vi "timed-delay-example.vi"() -> ()   [LabVIEW 2020]
uses:
  <vilib>/Platform/TimedLoop/XDataNode/timing_clust.ctl
  <vilib>/Platform/TimedLoop/XDataNode/nitl_modes.ctl
  <vilib>/Platform/TimedLoop/XDataNode/wakeup.ctl
  <vilib>/platform/TimedLoop/XDataNode/XDataNode.xnode
  <vilib>/Platform/TimedLoop/XDataNode/XDNodeRunTimeDep.lvlib
  <vilib>/measure/NI_MABase.lvlib
panel:
  out "Error out":errorcluster
  in  "Error":errorcluster
  out "Frame Duration":dbl
  in  "Delay between graphs(s)":dbl=1.0
  out "Waveform Graph":waveform(dbl)(graph)
  in  "Duration (s)":dbl=10.0
  in  "Samping rate (Sample/s)":dbl=10000.0
  in  "Frequency (Hz)":dbl=1000.0
  in  "Amplitude":dbl=1.0
  out "Waveform Graph":waveform(dbl)(graph)
  in  "Duration (s)":dbl=5.0
  in  "Samping rate (Sample/s)":dbl=1000.0
  in  "Frequency (Hz)":dbl=100.0
  in  "Amplitude":dbl=2.0
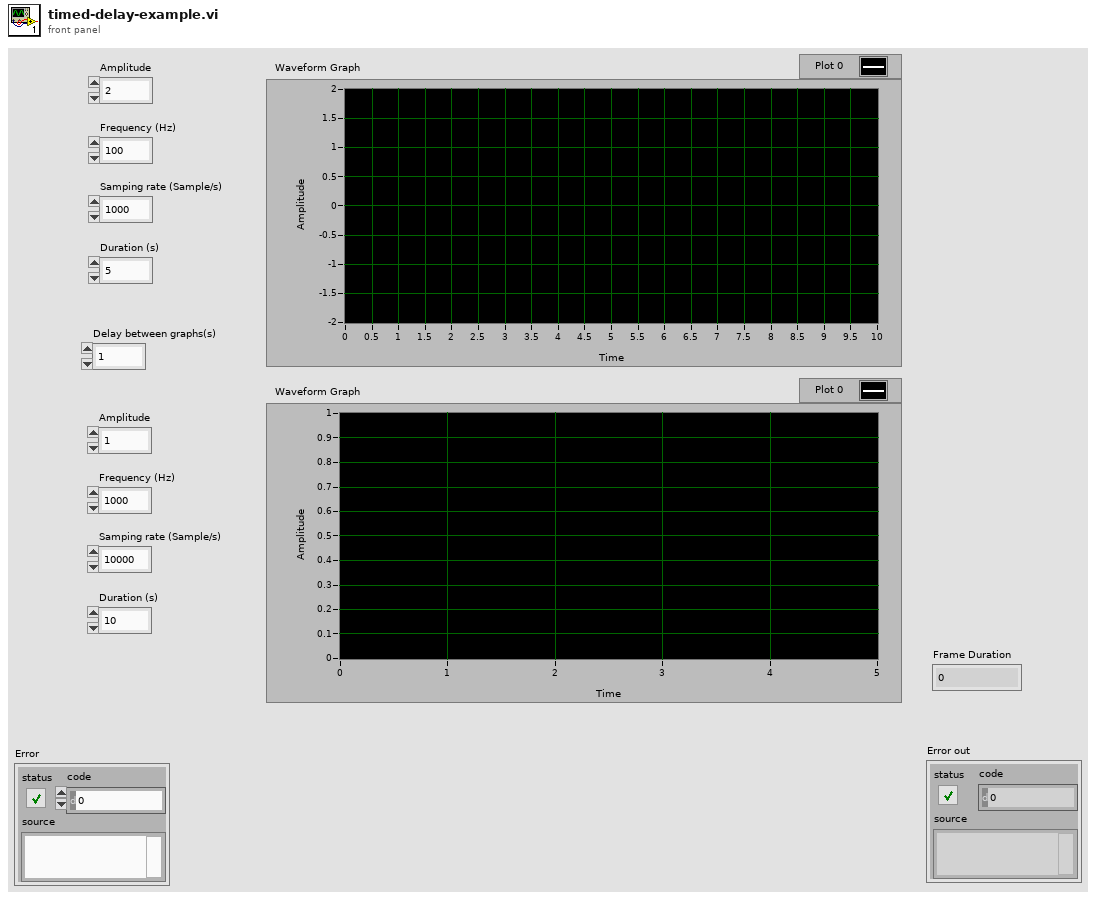
[diagram p1: front panel]
types:
  T1 = typedef "XDNodeRunTimeDep.lvlib/timing_clust.ctl" = cluster{"Expected End [f-1]":u64, "Actual End [f-1]":u64, "Finished Late? [f-1]":bool, "Expected End [i-1]":u64, "Actual End [i-1]":u64, "Finished Late? [i-1]":bool, "Expected Start [i]":u64, "Actual Start [i]":u64, "Expected Start [f]":u64, "Actual Start [f]":u64, "Source Name":string, "Structure Name":string, "Period":i64, "Deadline":i64, "Offset":i64, "Start":i64, "Priority":i32, "Timeout":i32, "Mode":T2, "Wakeup Reason":T3, "Error":errorcluster, "Source Type":string, "Secondary Source Type":string, "Global End Time":u64, "Global Start Time":u64, "Frame Duration":u64, "Iteration Duration":u64, "Assigned CPU":i32, "I/O Scan Engine Mode":u32}
  T2 = typedef "XDNodeRunTimeDep.lvlib/nitl_modes.ctl" = enum32{"No Change", "Process missed periods, maintain original phase", "Discard missed periods, maintain original phase", "Process missed periods, ignore original phase", "Discard missed periods, ignore original phase"}
  T3 = typedef "XDNodeRunTimeDep.lvlib/wakeup.ctl" = enum32{"Normal", "Aborted", "Asynchronous wakeup", "Timing source error", "Timed loop error", "Timeout"}
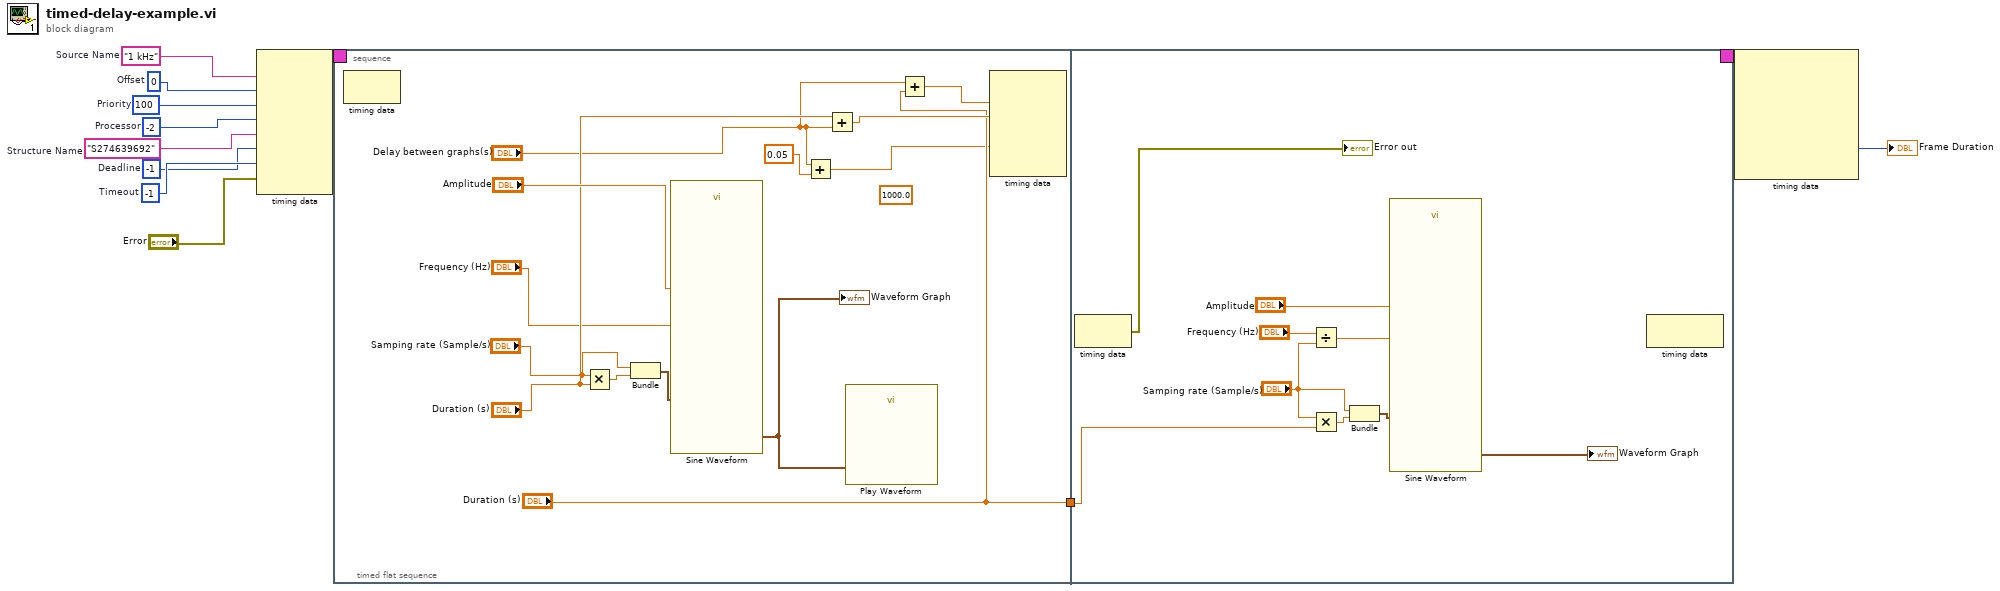
[diagram p0: block diagram]
diagram:
  w1 = "S274639692"  # Structure Name
  w2 = -2  # Processor
  w3 = 100  # Priority
  w4 = i64 0  # Offset
  w5 = "1 kHz"  # Source Name
  w6 = i64 -1  # Deadline
  w7 = -1  # Timeout
  n1 = node-c288(w5, w4, w3, w2, w1, w6, w7, "Error") -> (w11:T1)
  n2 = timed-sequence {
    timing: w11 -> [_]
    timing-out: [_] -> w10
    n3 = timed-flat-sequence {
      tunnel: ["Duration (s)"] -> w12
      tunnel: w12 -> [w34]
      frame #0 {
        (unwired) 1000.0 ("y")
        n4 = node-c288() -> ()  [unwired: 1 in, 1 out]
        n5 = Multiply(x="Samping rate (Sample/s)", y="Duration (s)") -> (x*y=w24:dbl)
        n6 = Bundle("Samping rate (Sample/s)"="Samping rate (Sample/s)", w24) -> (w25:cluster{"Samping rate (Sample/s)":dbl, dbl})  [unwired: 1 in]
        n7 = call <vilib>:"Sine Waveform.vi"("sampling info"=w25, "amplitude"="Amplitude", "frequency"="Frequency (Hz)") -> ("signal out"=w22:waveform(dbl))  [unwired: 7 in, 1 out]
        "Waveform Graph" <- w22
        n8 = Add(x="Delay between graphs(s)", y=0.05) -> (x+y=w14:dbl)
        n9 = Add(x="Duration (s)", y="Delay between graphs(s)") -> (x+y=w19:dbl)
        n10 = call "Play Waveform"("Data"=w22) -> ()  [unwired: 18 in, 1 out]
        n11 = Add(x="Delay between graphs(s)", y="Duration (s)") -> (x+y=w16:dbl)
        n12 = node-c288(w16, w19, w14) -> ()  [unwired: 3 in, 1 out]
      }
      frame #1 {
        n13 = node-c288() -> (→"Error out":errorcluster)  [unwired: 1 in]
        n14 = Divide(x="Frequency (Hz)", y="Samping rate (Sample/s)") -> (x/y=w36:dbl)
        n15 = Multiply(x="Samping rate (Sample/s)", y=w34) -> (x*y=w40:dbl)
        n16 = Bundle("Samping rate (Sample/s)"="Samping rate (Sample/s)", w40) -> (w37:cluster{"Samping rate (Sample/s)":dbl, dbl})  [unwired: 1 in]
        n17 = call <vilib>:"Sine Waveform.vi"("sampling info"=w37, "amplitude"="Amplitude", "frequency"=w36) -> ("signal out"=→"Waveform Graph":waveform(dbl))  [unwired: 7 in, 1 out]
        n18 = node-c288() -> ()  [unwired: 1 in, 1 out]
      }
    }
  }
  n19 = node-c288(w10) -> (→"Frame Duration":i64)  [unwired: 6 out]
